vi "Write Fill Orientation.vi"(8 "error in (no error)":errorcluster, 10 "Fill Orientation":u16(ring) items=["Horizontal", "Vertical"], 11 "Rectangle Settings in":refnum<class "Rectangle Settings.lvclass">) -> (0 "error out":errorcluster, 3 "Rectangle Settings out":refnum<class "Rectangle Settings.lvclass">)   [LabVIEW 2019, in "Rectangle Settings.lvclass"]
uses:
  Rectangle Settings.lvclass
  Rectangle Settings.lvclass/Rectangle Settings.ctl
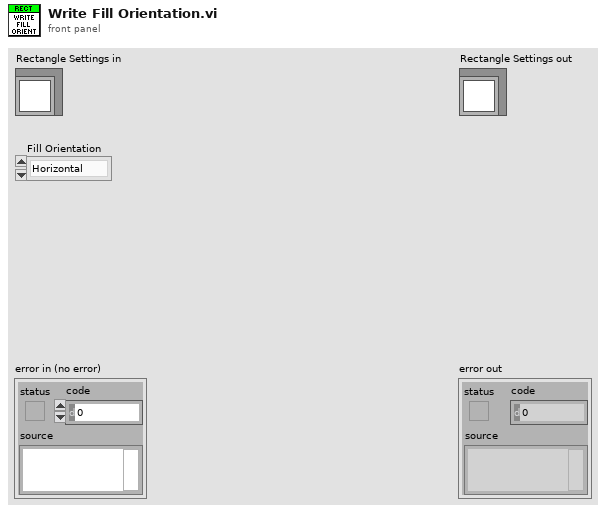
[diagram p1: front panel]
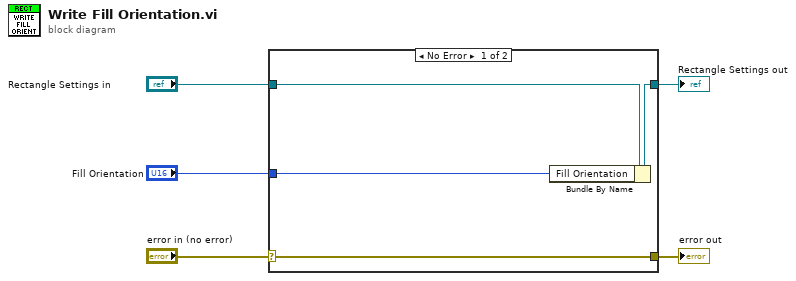
[diagram p0: block diagram]
diagram:
  n1 = case shown="No Error" "error in (no error)" {
    selector: "error in (no error)" -> [w9 w10]
    tunnel: [w9 w10] -> w4
    tunnel: [w7 w11] -> w2
    tunnel: "Rectangle Settings in" -> [w8 w11]
    tunnel: "Fill Orientation" -> [w6 _]
    frame No Error {
      n2 = Bundle By Name(cluster=w8, "Fill Orientation"=w6) -> (w7:refnum<class "Rectangle Settings.lvclass">)
    }
    frame Error {
    }
  }
  "error out" <- w4
  "Rectangle Settings out" <- w2
